vi "CRYASIOInitialize.vi"(8 "Sampling Rate":u32, 9 "Driver Name":string, 11 "error in (no error)":errorcluster) -> (0 "bResult":bool, 3 "error out":errorcluster)   [LabVIEW 2013]
uses:
  CRYASIO Global.vi
  CRY_ASIO.dll
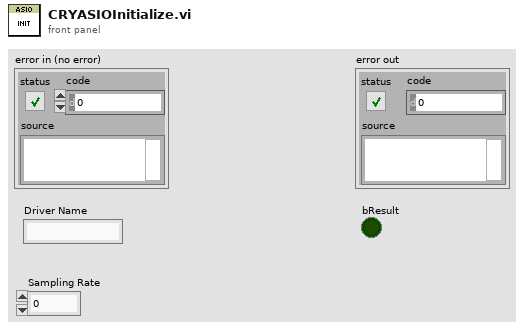
[diagram p1: front panel]
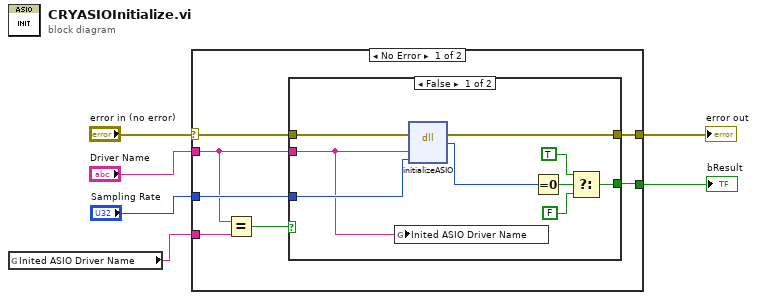
[diagram p0: block diagram]
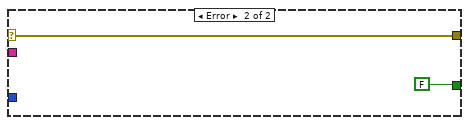
[diagram p3: hidden frame]
diagram:
  n1 = global read "CRYASIO Global.vi" "Inited ASIO Driver Name"() -> (w1:string)
  n2 = case shown="No Error" "error in (no error)" {
    selector: "error in (no error)" -> [w13 w26]
    tunnel: [w12 w26] -> w5
    tunnel: "Driver Name" -> [w8 _]
    tunnel: "Sampling Rate" -> [w11 _]
    tunnel: [w10 FALSE] -> w2
    tunnel: w1 -> [w9 _]
    frame No Error {
      n3 = Equal?(x=w8, y=w9) -> (x = y?=w7:bool)
      n4 = case shown="False" w7 {
        selector: w7 -> [_ w23]
        tunnel: w13 -> [w22 w24]
        tunnel: [w21 w24] -> w12
        tunnel: w11 -> [w20 _]
        tunnel: [w15 w23] -> w10
        tunnel: w8 -> [w14 _]
        frame False {
          n5 = global write "CRYASIO Global.vi" "Inited ASIO Driver Name"(w14) -> ()
          n6 = dll-call lib="D:/LabView_Project/CRY6181/CRY_ASIO.dll" fn="initializeASIO"(error in=w22, "arg1"=w14, "arg2"=w20) -> (error out=w21:errorcluster, "return type"=w18:i32)  [unwired: 4 in, 1 out]
          n7 = Equal To 0?(x=w18) -> (x = 0?=w19:bool)
          n8 = Select(t=TRUE, s=w19, f=FALSE) -> (s? t:f=w15:bool)
        }
        frame True {
        }
      }
    }
    frame Error {
    }
  }
  "error out" <- w5
  "bResult" <- w2
